vi "XML_to_array.vi"(0 "XML":string="<data><value>\n\n<struct>\n<member>\n<name>name</name>\n<value>intin</value>\n</member>\n<member>\n<name>value</name>\n<value><double>145.0</double></value>\n</member>\n<member>\n<name>action</name>\n<value>get</value>\n</member>\n</struct>\n\n</value></data>") -> (1 "ParsingErrors":string, 2 "Values":variant[](array[variant])=[variant(string "\n<member>\n<name>name</name>\n<value>intin</value>\n</member>\n<member>\n<name>value</name>\n<value><double>145.0</double></value>\n</member>\n<member>\n<name>action</name>\n<value>get</value>\n</member>\n")], 3 "Types":T1(array[ring])=[enum."struct"])   [LabVIEW 2010]
panel:
  out "Elements":string[](array[string])=["\n\n<struct>\n<member>\n<name>name</name>\n<value>intin</value>\n</member>\n<member>\n<name>value</name>\n<value><double>145.0</double></value>\n</member>\n<member>\n<name>action</name>\n<value>get</value>\n</member>\n</struct>\n\n"]
  out "RestOfElements":string
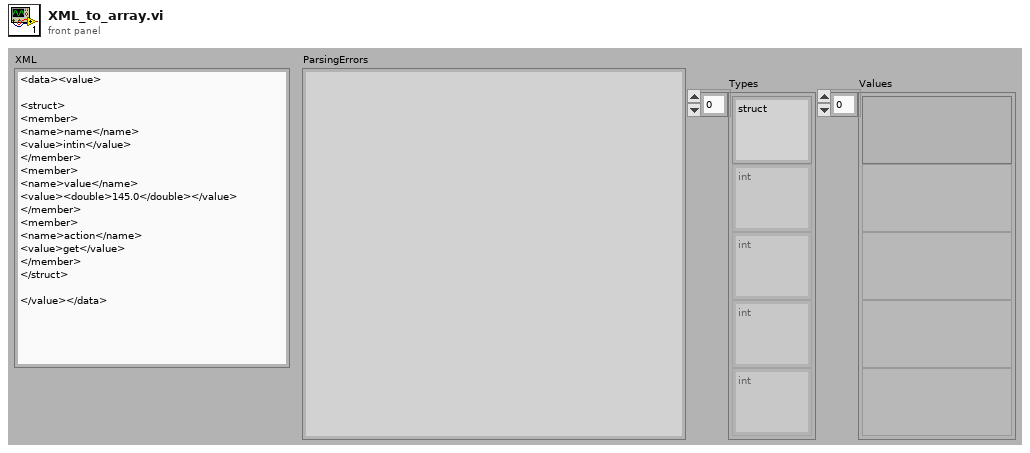
[diagram p1: front panel]
types:
  T1 = enum16{"int", "boolean", "string", "double", "dateTime", "base64", "struct", "array"}[]
  T2 = enum16{"int", "boolean", "string", "double", "dateTime", "base64", "struct", "array"}
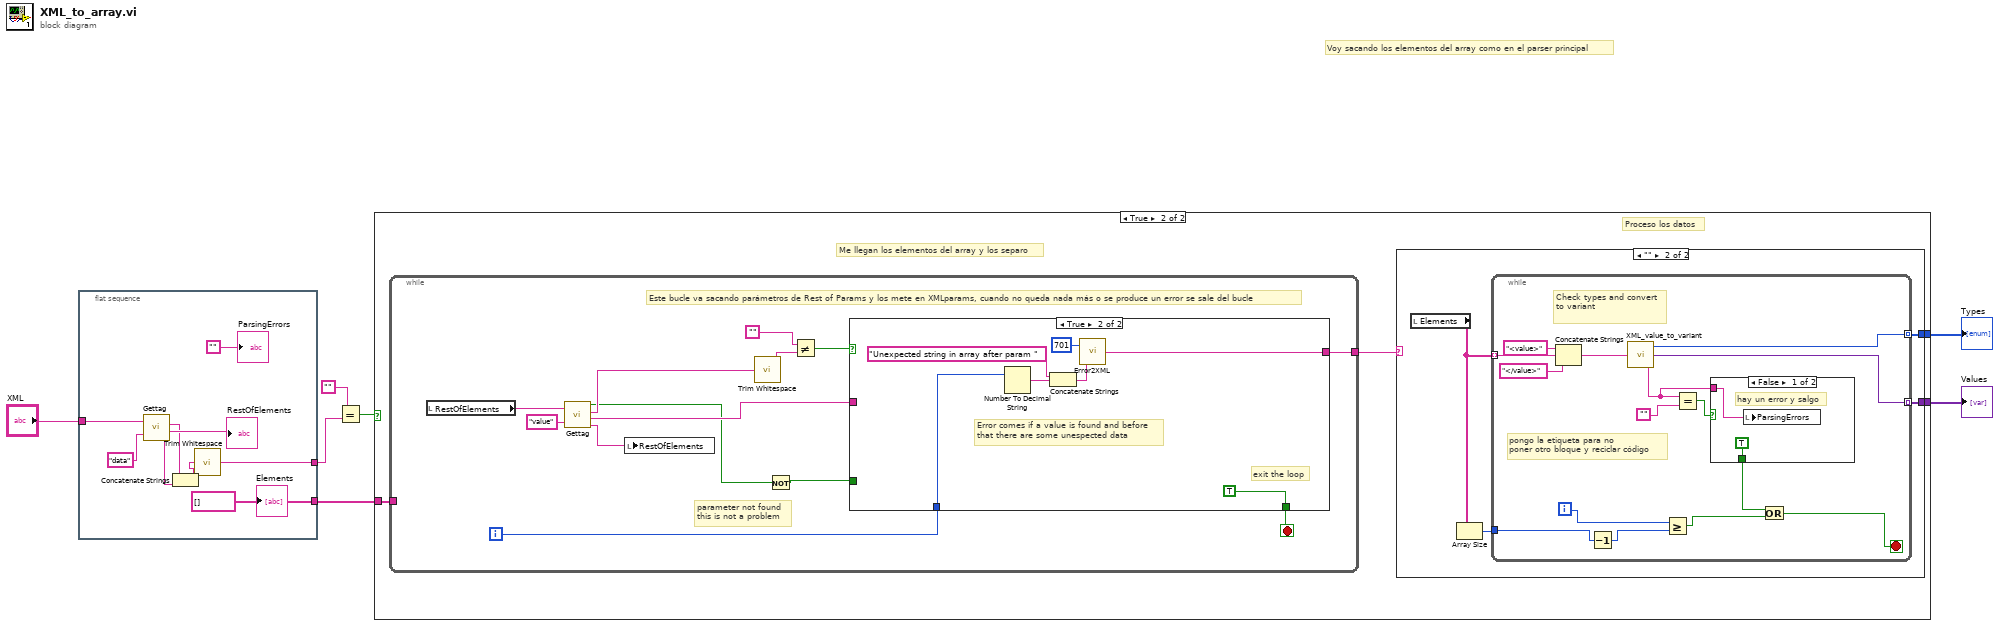
[diagram p0: block diagram]
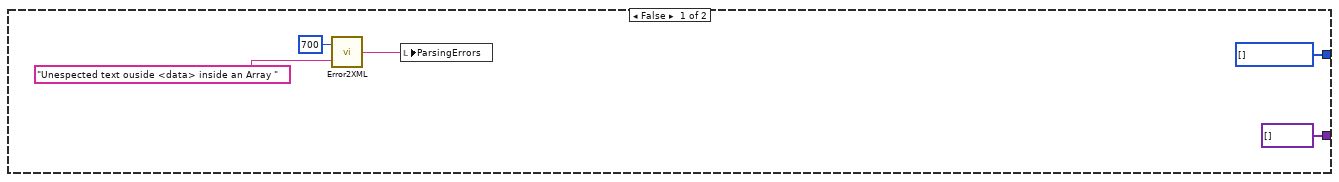
[diagram p2: hidden frame]
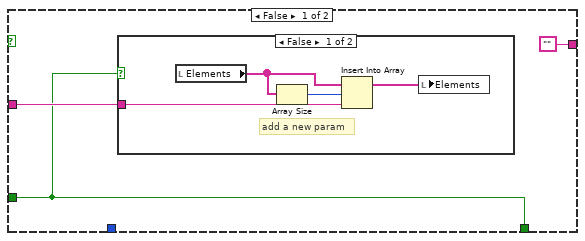
[diagram p3: hidden frame]
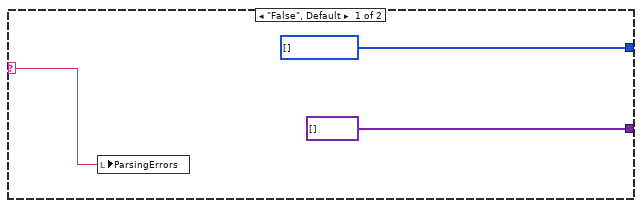
[diagram p5: hidden frame]
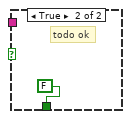
[diagram p6: hidden frame]
diagram:
  # "Voy sacando los elementos del array como en el parser principal"
  n1 = flat-sequence {
    tunnel: "XML" -> [w13]
    tunnel: [w16] -> w6
    tunnel: [w8] -> w2
    frame #0 {
      w16 = string[] [] ("XMLparams")
      n2 = call "Gettag.vi"("TagName"="data", "XML"=w13) -> ("AfterTag"=w10:string, "InsideTag"=→"RestOfElements":string, "BeforeTag"=w11:string)  [unwired: 1 out]
      n3 = Concatenate Strings(w11, w10) -> (w9:string)
      n4 = call <vilib>:"Trim Whitespace.vi"("string"=w9) -> ("trimmed string"=w8:string)  [unwired: 1 in]
      "Elements" <- w16
      "ParsingErrors" <- ""
    }
  }
  n5 = Equal?(x="", y=w2) -> (x = y?=w3:bool)
  n6 = case shown="True" w3 {
    tunnel: w6 -> [_ w25]
    tunnel: [w20 w23] -> w5
    tunnel: [variant[] [] w22] -> w4
    frame False {
      w20 = T1 [] items=["int", "boolean", "string", "double", "dateTime", "base64", "struct", "array"]
      n7 = call "Error2XML.vi"("FailDescriptor"="Unespected text ouside <data> inside an Array ", "FailID"=700) -> ("ErrorXML"=w19:string)
      n8 = local write "ParsingErrors"(w19) -> ()
    }
    frame True {
      # "Me llegan los elementos del array y los separo"
      # "Proceso los datos"
      n9 = while {
        tunnel: [w34] -> w24
        tunnel: w25 -> [_]
        i -> [w35]
        stop <- w33 stop-if-true
        # "Este bucle va sacando parámetros de Rest of Params y los mete en XMLparams, cuando no queda nada más o se produce un error se sale del bucle"
        # "parameter not found\nthis is not a problem"
        n10 = local read "RestOfElements"() -> (w31:string)
        n11 = call "Gettag.vi"("TagName"="value", "XML"=w31) -> ("AfterTag"=w29:string, "InsideTag"=w30:string, "BeforeTag"=w28:string, "Found?"=w26:bool)
        n12 = local write "RestOfElements"(w29) -> ()
        n13 = call <vilib>:"Trim Whitespace.vi"("string"=w28) -> ("trimmed string"=w37:string)  [unwired: 1 in]
        n14 = Not(x=w26) -> (.not. x?=w27:bool)
        n15 = Not Equal?(x="", y=w37) -> (x != y?=w36:bool)
        n16 = case shown="True" w36 {
          tunnel: w35 -> [_ w51]
          tunnel: ["" w48] -> w34
          tunnel: w27 -> [w39 _]
          tunnel: w30 -> [w40 _]
          tunnel: [w39 TRUE] -> w33
          frame False {
            n17 = case shown="False" w39 {
              tunnel: w40 -> [w44 _]
              frame False {
                # "add a new param"
                n18 = local read "Elements"() -> (w45:string[])
                n19 = Array Size(array=w45) -> (size(s)=w42:i32)
                n20 = Insert Into Array(array=w45, index=w42, new element=w44) -> (w43:string[])
                n21 = local write "Elements"(w43) -> ()
              }
              frame True {
              }
            }
          }
          frame True {
            # "Error comes if a value is found and before\nthat there are some unespected data"
            # "exit the loop"
            n22 = Number To Decimal String(number=w51) -> (decimal integer string=w50:string)  [unwired: 1 in]
            n23 = Concatenate Strings("Unexpected string in array after param " ("FailDescriptor"), w50) -> (w46:string)
            n24 = call "Error2XML.vi"("FailDescriptor"=w46, "FailID"=701) -> ("ErrorXML"=w48:string)
          }
        }
      }
      n25 = case shown="\"\"" w24 {
        selector: w24 -> [w53 _]
        tunnel: [w55 w59] -> w23
        tunnel: [variant[] [] w58] -> w22
        frame "False", Default {
          w55 = T1 [] items=["int", "boolean", "string", "double", "dateTime", "base64", "struct", "array"]
          n26 = local write "ParsingErrors"(w53) -> ()
        }
        frame "" {
          n27 = local read "Elements"() -> (w57:string[])
          n28 = Array Size(array=w57) -> (size(s)=w56:i32)
          n29 = while {
            tunnel: w57 -> [w61] mode=indexing
            tunnel: [w74] -> w59 mode=indexing
            tunnel: [w73] -> w58 mode=indexing
            tunnel: w56 -> [w64]
            i -> [w66]
            stop <- w67 stop-if-true
            # "pongo la etiqueta para no\nponer otro bloque y reciclar código"
            # "Check types and convert\nto variant"
            n30 = Concatenate Strings("<value>" ("string"), w61, "</value>" ("string")) -> (w60:string)
            n31 = Decrement(x=w64) -> (x-1=w65:i32)
            n32 = call "XML_value_to_variant.vi"("XML-param"=w60) -> ("ParsingErrors"=w68:string, "Value"=w73:variant, "Type"=w74:T2)
            n33 = Greater Or Equal?(x=w66, y=w65) -> (x >= y?=w72:bool)
            n34 = Equal?(x=w68, y="") -> (x = y?=w70:bool)
            n35 = case shown="False" w70 {
              tunnel: [TRUE FALSE] -> w69
              tunnel: w68 -> [w76 _]
              frame False {
                # "hay un error y salgo"
                n36 = local write "ParsingErrors"(w76) -> ()
              }
              frame True {
                # "todo ok"
              }
            }
            n37 = Or(x=w69, y=w72) -> (x .or. y?=w67:bool)
          }
        }
      }
    }
  }
  "Types" <- w5
  "Values" <- w4
